vi "StatusPub0MQ.vi"() -> (0 "error":errorcluster)   [LabVIEW 2012]
uses:
  <vilib>/addons/zeromq/zmq_context.lvclass
  <vilib>/addons/zeromq/zmq_socket.lvclass
  <vilib>/addons/zeromq/socket_type.ctl
  Global_Telescopio.vi
  <vilib>/addons/zeromq/zeromq.lvlib
panel:
  out "pulledCommand":string
  out "status":string
  out "time string":string
  in  "panelSstop":bool
  # "TCSPD STATUS PUB"
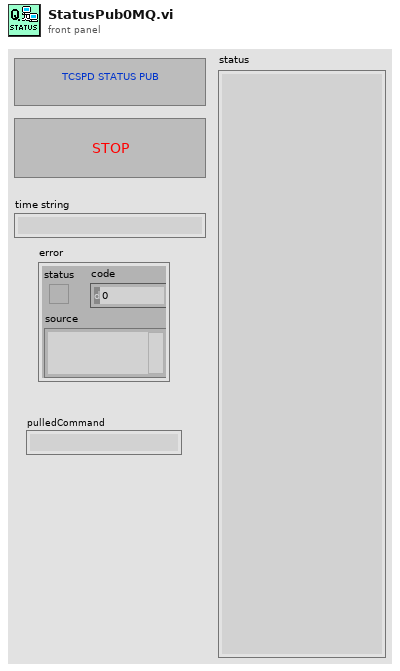
[diagram p1: front panel]
types:
  T1 = typedef "zeromq.lvlib/socket_type.ctl" = enum8{"ZMQ_PAIR", "ZMQ_PUB", "ZMQ_SUB", "ZMQ_REQ", "ZMQ_REP", "ZMQ_DEALER", "ZMQ_ROUTER", "ZMQ_PULL", "ZMQ_PUSH", "ZMQ_XPUB", "ZMQ_XSUB", "ZMQ_STREAM", "ZMQ_SERVER", "ZMQ_CLIENT", "ZMQ_RADIO", "ZMQ_DISH", "ZMQ_GATHER", "ZMQ_SCATTER", "ZMQ_DGRAM"}
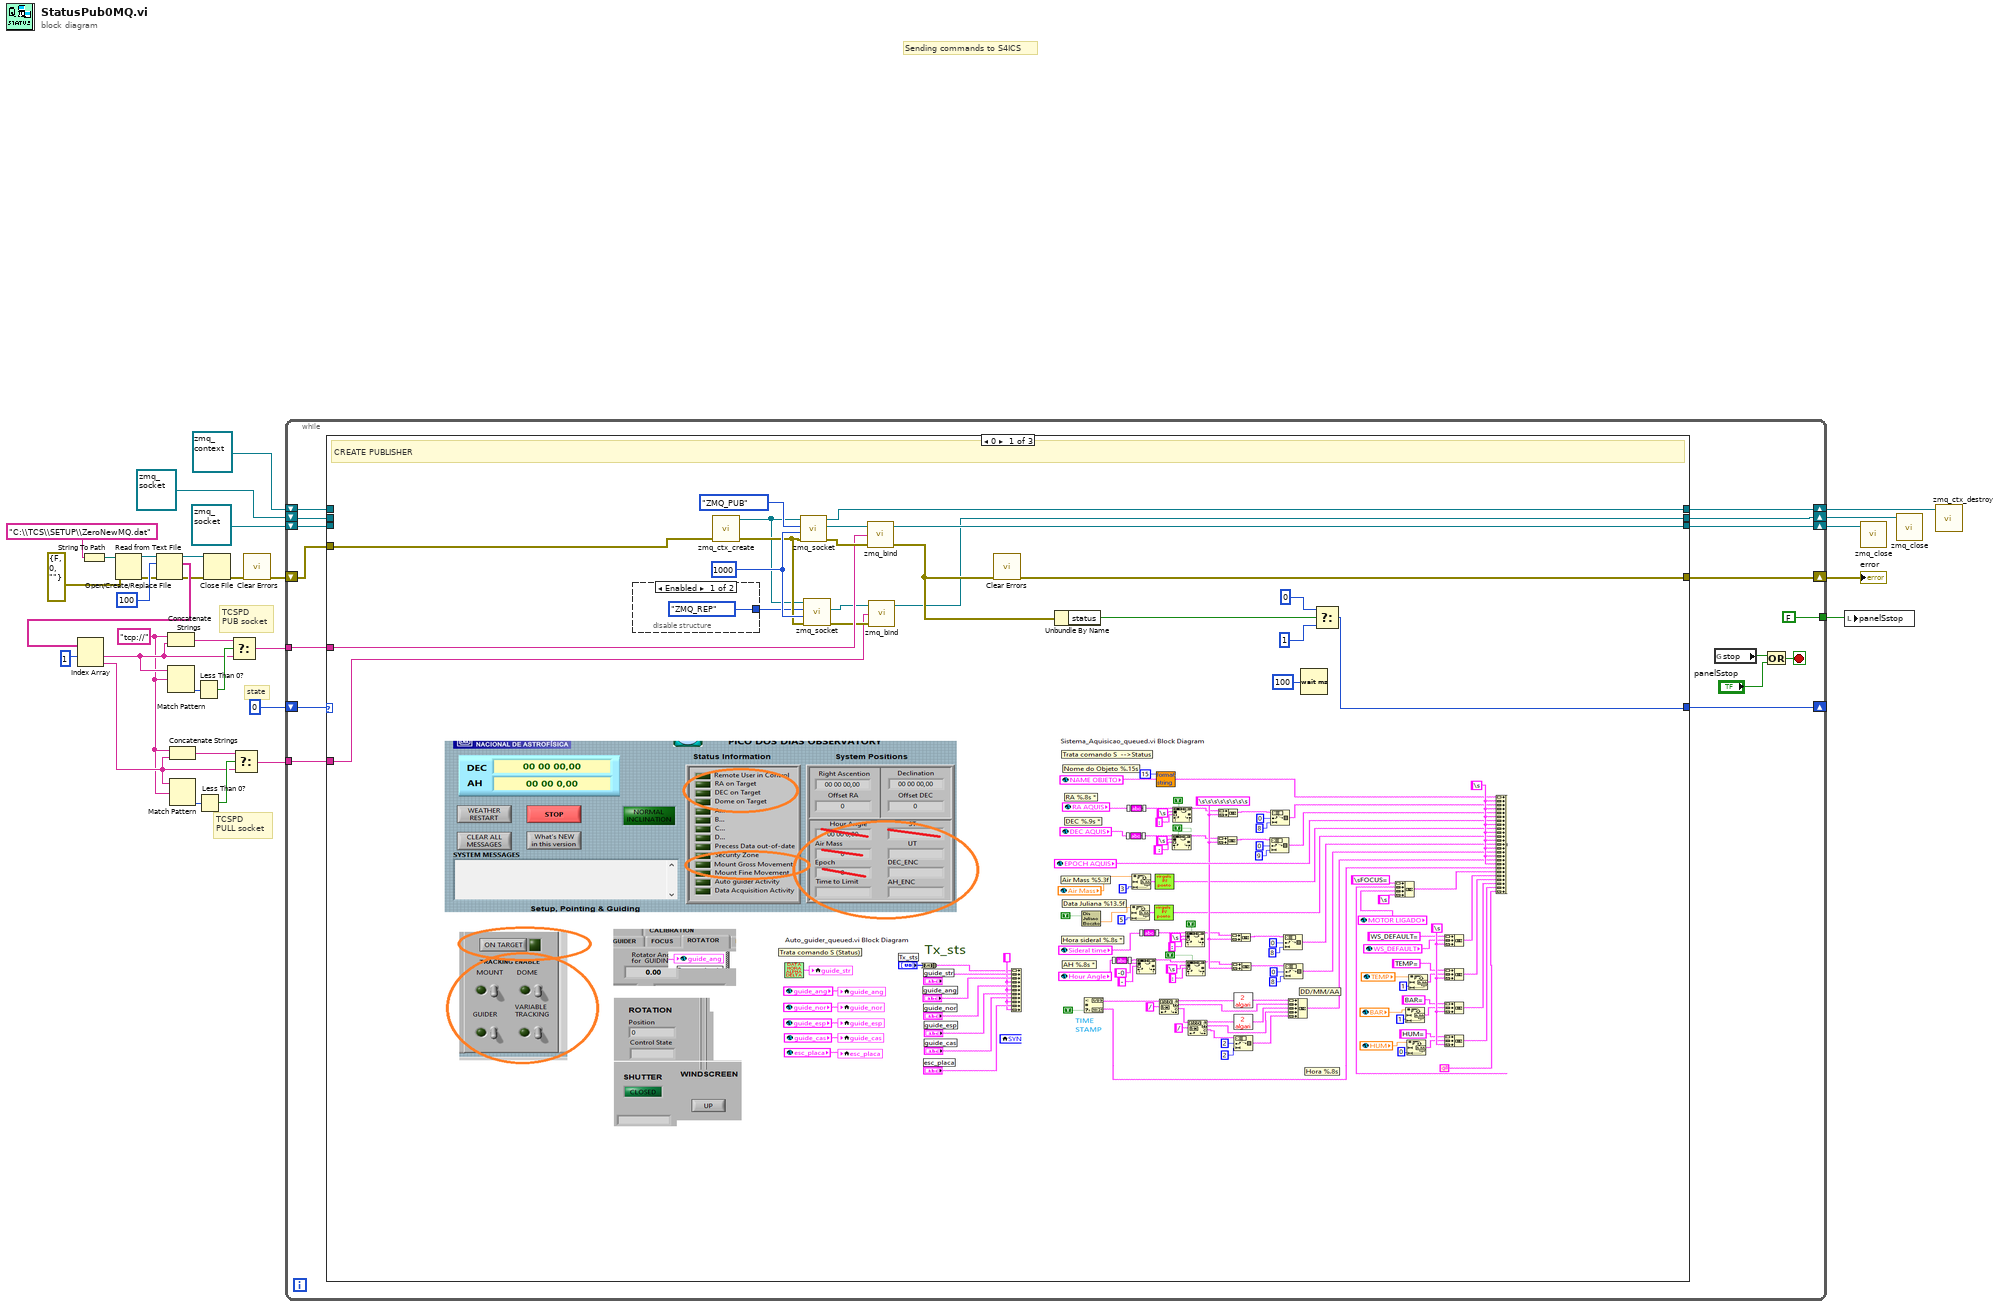
[diagram p0: block diagram]
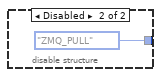
[diagram p2: hidden frame]
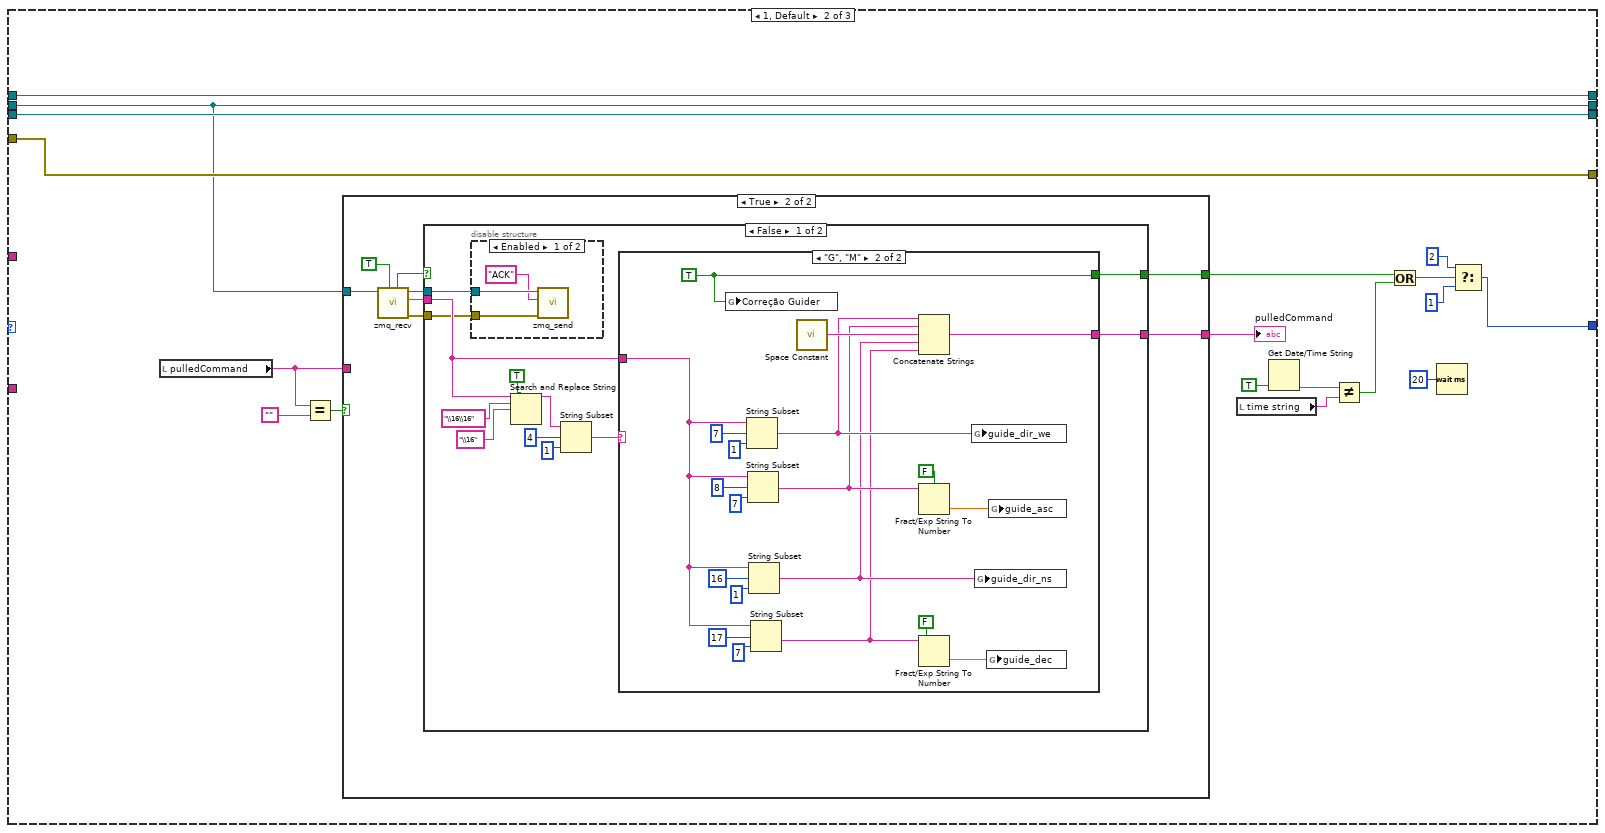
[diagram p3: hidden frame]
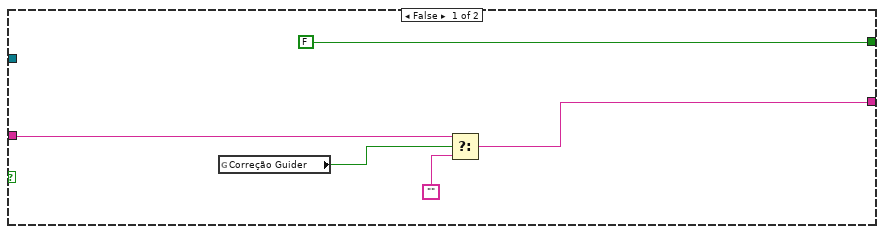
[diagram p4: hidden frame]
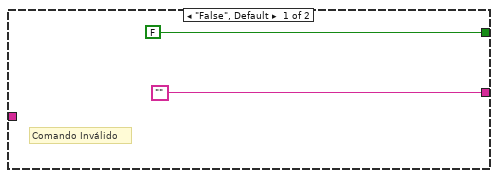
[diagram p6: hidden frame]
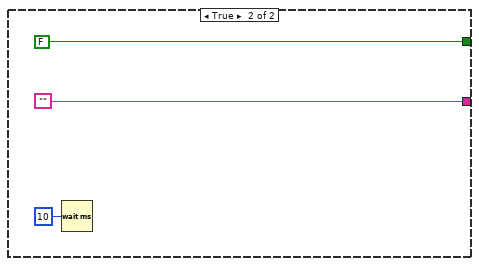
[diagram p7: hidden frame]
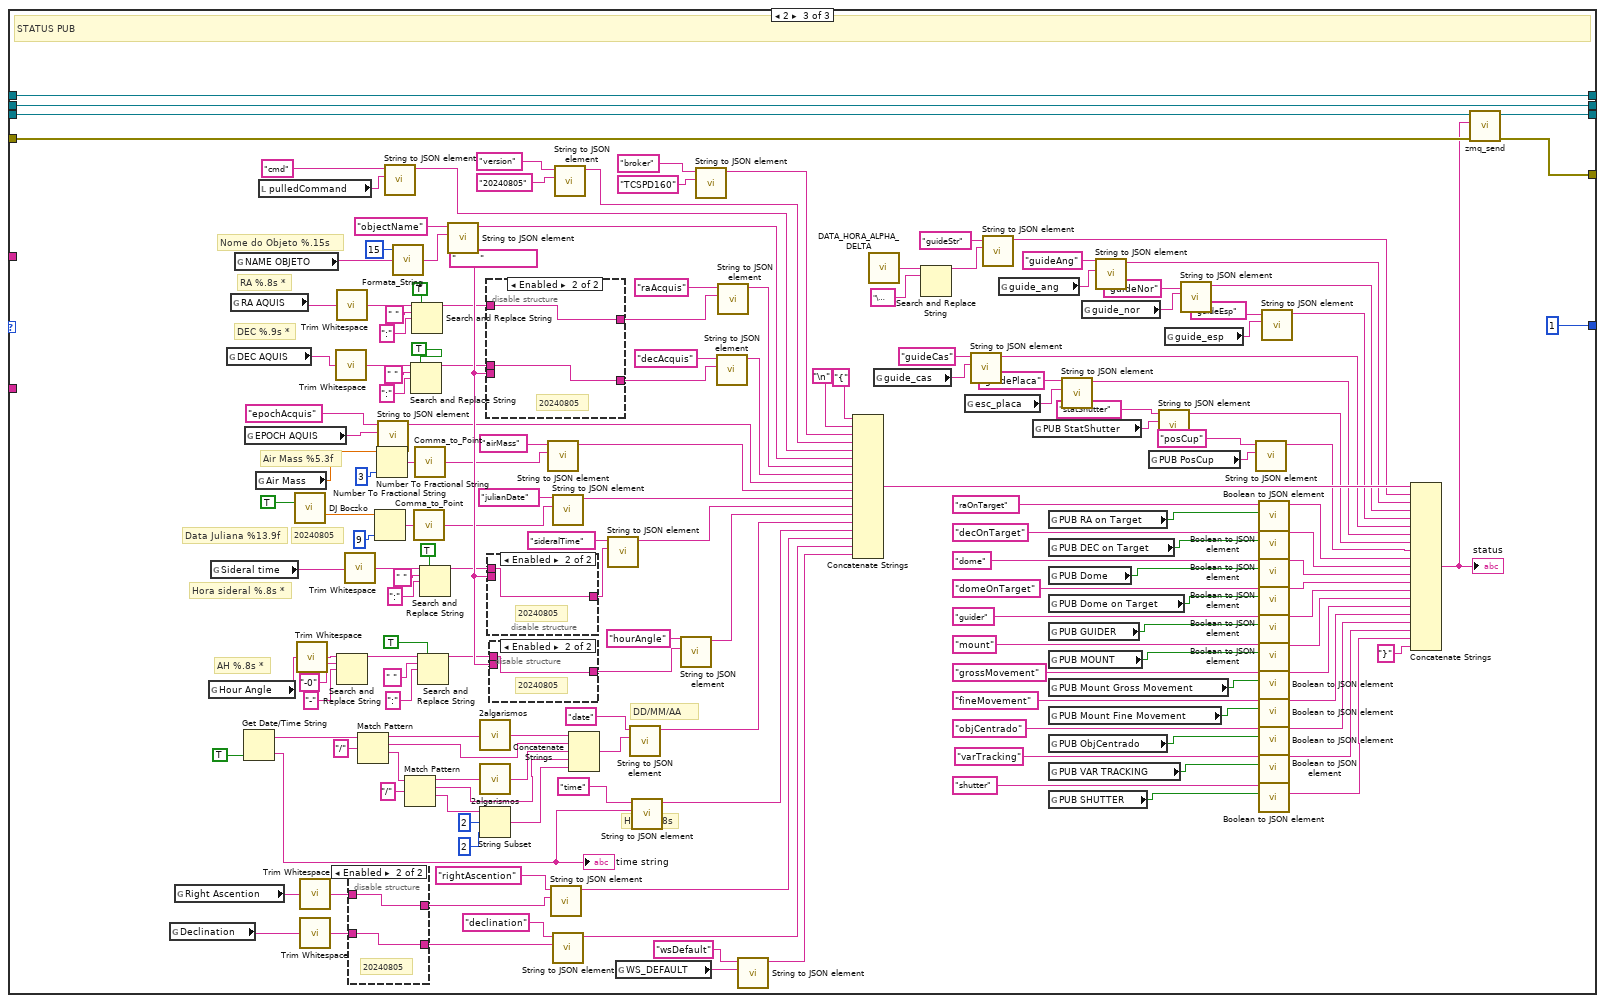
[diagram p8: hidden frame]
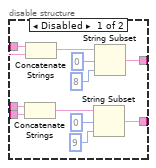
[diagram p9: hidden frame]
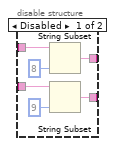
[diagram p10: hidden frame]
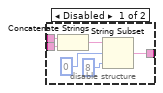
[diagram p11: hidden frame]
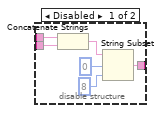
[diagram p12: hidden frame]
diagram:
  w2 = "tcp://"
  # "TCSPD\nPULL socket"
  # "TCSPD\nPUB socket"
  # "state"
  # "Sending commands to S4ICS"
  n1 = String To Path(string="C:\\TCS\\SETUP\\ZeroNewMQ.dat") -> (path=w31:path)
  n2 = Open/Create/Replace File(file path (use dialog)=w31, error in=errorcluster {"status"=FALSE, "code"=0, "source"=""}) -> (refnum out=w29:refnum<file>, error out=w22:errorcluster)  [unwired: 4 in, 1 out]
  n3 = Read from Text File(file (use dialog)=w29, count=100, error in=w22) -> (refnum out=w25:refnum<file>, text=w27:string[], error out=w19:errorcluster)  [unwired: 1 in, 1 out]
  n4 = Index Array(array=w27, index #1=1 ("index")) -> (element #1=w11:string, element #2=w3:string)  [unwired: 1 in]
  n5 = Concatenate Strings(w2, w11) -> (w13:string)
  n6 = Match Pattern(string=w11, regular expression=w2) -> (offset past match=w12:i32)  [unwired: 1 in, 3 out]
  n7 = Concatenate Strings(w2, w3) -> (w5:string)
  n8 = Match Pattern(string=w3, regular expression=w2) -> (offset past match=w6:i32)  [unwired: 1 in, 3 out]
  n9 = Less Than 0?(x=w12) -> (x < 0?=w14:bool)
  n10 = Less Than 0?(x=w6) -> (x < 0?=w4:bool)
  n11 = Close File(refnum=w25, error in=w19) -> (error out=w20:errorcluster)  [unwired: 1 out]
  n12 = Select(t=w13, s=w14, f=w11) -> (s? t:f=w10:string)
  n13 = Select(t=w5, s=w4, f=w3) -> (s? t:f=w1:string)
  n14 = call <vilib>:"Clear Errors.vi"("error in (no error)"=w20) -> ("error out"=w18:errorcluster)  [unwired: 6 in]
  n15 = while {
    shift-right: [w46] -> _
    shift-left: u16 0 -> [w48]
    tunnel: w10 -> [w44]
    shift-right: [w42] -> w16
    shift-left: refnum<class "zmq_socket.lvclass"> refnum ("socket out") -> [w43]
    shift-right: [w41] -> w21
    shift-left: refnum<class "zmq_context.lvclass"> refnum ("context out") -> [w40]
    tunnel: [FALSE] -> w15
    shift-right: [w37] -> w9
    shift-left: w18 -> [w47]
    shift-right: [w35] -> w7
    shift-left: refnum<class "zmq_socket.lvclass"> refnum ("socket out") -> [w34]
    tunnel: w1 -> [w33]
    stop <- w45 stop-if-true
    n16 = case shown="0" w48 {
      tunnel: w47 -> [w66 w87 w311]
      tunnel: [w68 w88 u16 1] -> w46
      tunnel: w44 -> [w59 _ _]
      tunnel: w43 -> [_ w86 w314]
      tunnel: [w58 w86 w313] -> w42
      tunnel: [w67 w84 w312] -> w41
      tunnel: w40 -> [_ w84 w312]
      tunnel: [w61 w87 w310] -> w37
      tunnel: [w50 w85 w309] -> w35
      tunnel: w34 -> [_ w85 w309]
      tunnel: w33 -> [w49 _ _]
      frame 0 {
        w56 = 1000 ("linger (ms)")
        # "CREATE PUBLISHER"
        n17 = disable-structure shown="Enabled" {
          disable-tunnel: [socket_type."ZMQ_REP" ("socket type") socket_type."ZMQ_PULL" ("socket type")] -> w53
          frame Enabled {
          }
          frame Disabled {
          }
        }
        n18 = call <vilib>:"zmq_ctx_create.vi"("error in"=w66) -> ("error out"=w55:errorcluster, "context out"=w54:refnum<class "zmq_context.lvclass">)  [unwired: 3 in]
        n19 = call <vilib>:"zmq_socket.vi"("error in"=w55, "linger (ms)"=w56, "socket type"=socket_type."ZMQ_PUB", "context in"=w54) -> ("error out"=w63:errorcluster, "socket out"=w64:refnum<class "zmq_socket.lvclass">, "context out"=w67:refnum<class "zmq_context.lvclass">)  [unwired: 1 in]
        n20 = call <vilib>:"zmq_socket.vi"("error in"=w55, "linger (ms)"=w56, "socket type"=w53, "context in"=w54) -> ("error out"=w51:errorcluster, "socket out"=w52:refnum<class "zmq_socket.lvclass">)  [unwired: 1 in, 1 out]
        n21 = call <vilib>:"zmq_bind.vi"("error in"=w63, "endpoint"=w59, "socket in"=w64) -> ("error out"=w60:errorcluster, "socket out"=w58:refnum<class "zmq_socket.lvclass">)  [unwired: 1 in]
        n22 = call <vilib>:"zmq_bind.vi"("error in"=w51, "endpoint"=w49, "socket in"=w52) -> ("socket out"=w50:refnum<class "zmq_socket.lvclass">)  [unwired: 1 in, 1 out]
        n23 = call <vilib>:"Clear Errors.vi"("error in (no error)"=w60) -> ("error out"=w61:errorcluster)  [unwired: 6 in]
        n24 = Unbundle By Name(w60) -> ("status"=w57:bool)
        n25 = Wait (ms)(milliseconds to wait=u32 100) -> ()  [unwired: 1 out]
        n26 = Select(t=u16 0, s=w57, f=u16 1) -> (s? t:f=w68:u16)
      }
      frame 1, Default {
        n27 = local read "pulledCommand"() -> (w76:string)
        n28 = Equal?(x=w76, y="") -> (x = y?=w78:bool)
        n29 = case shown="True" w78 {
          tunnel: w85 -> [_ w103]
          tunnel: [w91 w100] -> w73
          tunnel: w76 -> [w93 _]
          tunnel: [FALSE w99] -> w75
          frame False {
            n30 = global read "Global_Telescopio.vi" "Correção Guider"() -> (w94:bool)
            n31 = Select(t=w93, s=w94, f="") -> (s? t:f=w91:string)
          }
          frame True {
            n32 = call <vilib>:"zmq_recv.vi"("no block? (F)"=TRUE, "socket in"=w103) -> ("error out"=w96:errorcluster, "data"=w101:string, "socket out"=w97:refnum<class "zmq_socket.lvclass">, "timeout?"=w98:bool)  [unwired: 3 in, 1 out]
            n33 = case shown="False" w98 {
              tunnel: w101 -> [w108 _]
              tunnel: [w107 ""] -> w100
              tunnel: [w106 FALSE] -> w99
              tunnel: w97 -> [w105 _]
              tunnel: w96 -> [w104 _]
              frame False {
                n34 = disable-structure shown="Enabled" {
                  disable-tunnel: w105 -> [w118 _]
                  disable-tunnel: w104 -> [w117 _]
                  frame Enabled {
                    n35 = call <vilib>:"zmq_send.vi"("error in"=w117, "data"="ACK", "socket in"=w118) -> ()  [unwired: 4 in, 2 out]
                  }
                  frame Disabled {
                  }
                }
                n36 = Search and Replace String(replace all?=TRUE ("replace all? (F)"), input string=w108, search string="\\16\\16", replace string="\\16" ("replace string (\"\")")) -> (result string=w110:string)  [unwired: 4 in, 3 out]
                n37 = String Subset(string=w110, offset (0)=4, length (rest)=1 ("length (rest)")) -> (substring=w109:string)
                n38 = case shown="\"G\", \"M\"" w109 {
                  tunnel: w108 -> [_ w127]
                  tunnel: ["" w121] -> w107
                  tunnel: [FALSE w128] -> w106
                  frame "False", Default {
                    # "Comando Inválido"
                  }
                  frame "G", "M" {
                    w128 = TRUE ("replace all? (F)")
                    n39 = global write "Global_Telescopio.vi" "Correção Guider"(w128) -> ()
                    n40 = String Subset(string=w127, offset (0)=7, length (rest)=1 ("length (rest)")) -> (substring=w125:string)
                    n41 = String Subset(string=w127, offset (0)=8, length (rest)=7 ("length (rest)")) -> (substring=w124:string)
                    n42 = String Subset(string=w127, offset (0)=16, length (rest)=1 ("length (rest)")) -> (substring=w123:string)
                    n43 = String Subset(string=w127, offset (0)=17, length (rest)=7 ("length (rest)")) -> (substring=w122:string)
                    n44 = call <vilib>:"Space Constant.vi"() -> ("String"=w126:string)
                    n45 = Concatenate Strings(w125, w124, w126, w123, w122) -> (w121:string)
                    n46 = Fract/Exp String To Number(use system decimal point (T)=FALSE, string=w124) -> (number=w139:dbl)  [unwired: 2 in, 1 out]
                    n47 = Fract/Exp String To Number(use system decimal point (T)=FALSE, string=w122) -> (number=w140:dbl)  [unwired: 2 in, 1 out]
                    n48 = global write "Global_Telescopio.vi" "guide_dir_we"(w125) -> ()
                    n49 = global write "Global_Telescopio.vi" "guide_dir_ns"(w123) -> ()
                    n50 = global write "Global_Telescopio.vi" "guide_dec"(w140) -> ()
                    n51 = global write "Global_Telescopio.vi" "guide_asc"(w139) -> ()
                  }
                }
              }
              frame True {
                n52 = Wait (ms)(milliseconds to wait=u32 10) -> ()  [unwired: 1 out]
              }
            }
          }
        }
        "pulledCommand" <- w73
        n53 = local read "time string"() -> (w79:string)
        n54 = Get Date/Time String(want seconds? (F)=TRUE) -> (time string=w80:string)  [unwired: 2 in, 1 out]
        n55 = Not Equal?(x=w80, y=w79) -> (x != y?=w82:bool)
        n56 = Or(x=w75, y=w82) -> (x .or. y?=w83:bool)
        n57 = Wait (ms)(milliseconds to wait=u32 20) -> ()  [unwired: 1 out]
        n58 = Select(t=u16 2, s=w83, f=u16 1) -> (s? t:f=w88:u16)
      }
      frame 2 {
        w285 = "        " ("string")
        # "20240805"
        # "Hora %.8s"
        # "DD/MM/AA"
        # "AH %.8s *"
        # "Hora sideral %.8s *"
        # "Data Juliana %13.9f"
        # "Air Mass %5.3f"
        # "DEC %.9s *"
        # "RA %.8s *"
        # "Nome do Objeto %.15s"
        # "STATUS PUB"
        n59 = global read "Global_Telescopio.vi" "Declination"() -> (w170:string)
        n60 = global read "Global_Telescopio.vi" "Right Ascention"() -> (w168:string)
        n61 = global read "Global_Telescopio.vi" "Hour Angle"() -> (w308:string)
        n62 = global read "Global_Telescopio.vi" "Sideral time"() -> (w280:string)
        n63 = global read "Global_Telescopio.vi" "DEC AQUIS"() -> (w269:string)
        n64 = global read "Global_Telescopio.vi" "RA AQUIS"() -> (w259:string)
        n65 = global read "Global_Telescopio.vi" "NAME OBJETO"() -> (w302:string)
        n66 = Get Date/Time String(want seconds? (F)=TRUE) -> (date string=w318:string, time string=w316:string)  [unwired: 2 in]
        "time string" <- w316
        n67 = global read "Global_Telescopio.vi" "EPOCH AQUIS"() -> (w248:string)
        n68 = global read "Global_Telescopio.vi" "Air Mass"() -> (w301:dbl)
        n69 = local read "pulledCommand"() -> (w152:string)
        n70 = call "DJ Boczko.vi"("TRUE = Hora Local\nFALSE = UT"=TRUE ("TRUE = Hora Local\nFALSE = UT")) -> ("Dia Juliano"=w274:dbl)  [unwired: 6 in, 8 out]
        n71 = call <vilib>:"Trim Whitespace.vi"("string"=w308) -> ("trimmed string"=w307:string)  [unwired: 1 in]
        n72 = call <vilib>:"Trim Whitespace.vi"("string"=w168) -> ("trimmed string"=w167:string)  [unwired: 1 in]
        n73 = call <vilib>:"Trim Whitespace.vi"("string"=w170) -> ("trimmed string"=w169:string)  [unwired: 1 in]
        n74 = call <vilib>:"Trim Whitespace.vi"("string"=w269) -> ("trimmed string"=w268:string)  [unwired: 1 in]
        n75 = call <vilib>:"Trim Whitespace.vi"("string"=w259) -> ("trimmed string"=w260:string)  [unwired: 1 in]
        n76 = Search and Replace String(input string=w307, search string="-0", replace string="-" ("replace string (\"\")")) -> (result string=w306:string)  [unwired: 5 in, 3 out]
        n77 = call <vilib>:"Trim Whitespace.vi"("string"=w280) -> ("trimmed string"=w279:string)  [unwired: 1 in]
        n78 = disable-structure shown="Enabled" {
          disable-tunnel: w169 -> [w337 w338]
          disable-tunnel: w167 -> [w335 w339]
          disable-tunnel: [w334 w339] -> w161
          disable-tunnel: [w333 w338] -> w160
          frame Disabled {
            n79 = String Subset(string=w335, length (rest)=8 ("length (rest)")) -> (substring=w334:string)  [unwired: 1 in]
            n80 = String Subset(string=w337, length (rest)=9 ("length (rest)")) -> (substring=w333:string)  [unwired: 1 in]
          }
          frame Enabled {
            # "20240805"
          }
        }
        n81 = Match Pattern(string=w318, regular expression="/") -> (before substring=w289:string, match substring=w295:string, after substring=w288:string)  [unwired: 1 in, 1 out]
        n82 = Number To Fractional String(number=w274, precision (6)=i16 9) -> (F-format string=w275:string)  [unwired: 2 in]
        n83 = Number To Fractional String(number=w301, precision (6)=i16 3) -> (F-format string=w272:string)  [unwired: 2 in]
        n84 = call "String to JSON element.vi"("value"=w248, "keyword"="epochAcquis") -> ("JSON element"=w247:string)  [unwired: 8 in, 1 out]
        n85 = call "String to JSON element.vi"("value"=w152, "keyword"="cmd") -> ("JSON element"=w147:string)  [unwired: 8 in, 1 out]
        n86 = call "Formata_String.vi"("entrada"=w302, "Num de Caracteres"=15) -> ("saida"=w257:string)  [unwired: 3 in]
        n87 = Match Pattern(string=w288, regular expression="/") -> (before substring=w290:string, match substring=w297:string, after substring=w291:string)  [unwired: 1 in, 1 out]
        n88 = Search and Replace String(replace all?=TRUE ("replace all? (F)"), input string=w268, search string=" ", replace string=":" ("replace string (\"\")")) -> (result string=w265:string)  [unwired: 4 in, 3 out]
        n89 = Search and Replace String(replace all?=TRUE ("replace all? (F)"), input string=w260, search string=" ", replace string=":" ("replace string (\"\")")) -> (result string=w264:string)  [unwired: 4 in, 3 out]
        n90 = call "Comma_to_Point.vi"("Lat_A"=w275) -> ("Saída"=w242:string)
        n91 = call "Comma_to_Point.vi"("Lat_A"=w272) -> ("Saída"=w246:string)
        n92 = Search and Replace String(replace all?=TRUE ("replace all? (F)"), input string=w306, search string=" ", replace string=":" ("replace string (\"\")")) -> (result string=w284:string)  [unwired: 4 in, 3 out]
        n93 = Search and Replace String(replace all?=TRUE ("replace all? (F)"), input string=w279, search string=" ", replace string=":" ("replace string (\"\")")) -> (result string=w276:string)  [unwired: 4 in, 3 out]
        n94 = call "String to JSON element.vi"("value"=w257, "keyword"="objectName") -> ("JSON element"=w256:string)  [unwired: 8 in, 1 out]
        n95 = call "2algarismos.vi"("entrada"=w289) -> ("saida"=w294:string)
        n96 = call "2algarismos.vi"("entrada"=w290) -> ("saida"=w296:string)
        n97 = String Subset(string=w291, offset (0)=2, length (rest)=2 ("length (rest)")) -> (substring=w298:string)
        n98 = disable-structure shown="Enabled" {
          disable-tunnel: w285 -> [w329 _]
          disable-tunnel: w265 -> [w326 w331]
          disable-tunnel: w264 -> [w323 w330]
          disable-tunnel: [w320 w330] -> w255
          disable-tunnel: [w319 w331] -> w252
          frame Disabled {
            n99 = Concatenate Strings(w326, w329) -> (w325:string)
            n100 = Concatenate Strings(w323, w329) -> (w324:string)
            n101 = String Subset(string=w325, offset (0)=0, length (rest)=9 ("length (rest)")) -> (substring=w319:string)
            n102 = String Subset(string=w324, offset (0)=0, length (rest)=8 ("length (rest)")) -> (substring=w320:string)
          }
          frame Enabled {
            # "20240805"
          }
        }
        n103 = disable-structure shown="Enabled" {
          disable-tunnel: w285 -> [w352 _]
          disable-tunnel: w276 -> [w349 w353]
          disable-tunnel: [w347 w353] -> w239
          frame Disabled {
            n104 = Concatenate Strings(w349, w352) -> (w348:string)
            n105 = String Subset(string=w348, offset (0)=0, length (rest)=8 ("length (rest)")) -> (substring=w347:string)
          }
          frame Enabled {
            # "20240805"
          }
        }
        n106 = disable-structure shown="Enabled" {
          disable-tunnel: w285 -> [w345 _]
          disable-tunnel: w284 -> [w343 w346]
          disable-tunnel: [w340 w346] -> w236
          frame Disabled {
            n107 = Concatenate Strings(w343, w345) -> (w344:string)
            n108 = String Subset(string=w344, offset (0)=0, length (rest)=8 ("length (rest)")) -> (substring=w340:string)
          }
          frame Enabled {
            # "20240805"
          }
        }
        n109 = call "String to JSON element.vi"("value"=w246, "keyword"="airMass") -> ("JSON element"=w244:string)  [unwired: 8 in, 1 out]
        n110 = call "String to JSON element.vi"("value"=w161, "keyword"="rightAscention") -> ("JSON element"=w159:string)  [unwired: 8 in, 1 out]
        n111 = call "String to JSON element.vi"("value"=w242, "keyword"="julianDate") -> ("JSON element"=w241:string)  [unwired: 8 in, 1 out]
        n112 = call "String to JSON element.vi"("value"=w160, "keyword"="declination") -> ("JSON element"=w158:string)  [unwired: 8 in, 1 out]
        n113 = call "String to JSON element.vi"("value"="20240805", "keyword"="version") -> ("JSON element"=w148:string)  [unwired: 8 in, 1 out]
        n114 = Concatenate Strings(w294, w295, w296, w297, w298) -> (w233:string)
        n115 = call "String to JSON element.vi"("value"=w239, "keyword"="sideralTime") -> ("JSON element"=w238:string)  [unwired: 8 in, 1 out]
        n116 = global read "Global_Telescopio.vi" "WS_DEFAULT"() -> (w145:string)
        n117 = call "String to JSON element.vi"("value"=w233, "keyword"="date") -> ("JSON element"=w232:string)  [unwired: 8 in, 1 out]
        n118 = call "String to JSON element.vi"("value"=w316, "keyword"="time") -> ("JSON element"=w230:string)  [unwired: 8 in, 1 out]
        n119 = call "String to JSON element.vi"("value"=w236, "keyword"="hourAngle") -> ("JSON element"=w235:string)  [unwired: 8 in, 1 out]
        n120 = call "String to JSON element.vi"("value"="TCSPD160", "keyword"="broker") -> ("JSON element"=w149:string)  [unwired: 8 in, 1 out]
        n121 = call "String to JSON element.vi"("value"=w252, "keyword"="decAcquis") -> ("JSON element"=w250:string)  [unwired: 8 in, 1 out]
        n122 = call "String to JSON element.vi"("value"=w255, "keyword"="raAcquis") -> ("JSON element"=w253:string)  [unwired: 8 in, 1 out]
        n123 = call "String to JSON element.vi"("value"=w145, "keyword"="wsDefault") -> ("JSON element"=w144:string)  [unwired: 8 in, 1 out]
        n124 = Concatenate Strings("{", "\n", w149, w148, w147, w256, w253, w250, w247, w244, w241, w238, w235, w232, w230, w159, w158, w144) -> (w192:string)
        n125 = call "DATA_HORA_ALPHA_DELTA.vi"() -> ("SAIDA"=w166:string)  [unwired: 2 in]
        n126 = global read "Global_Telescopio.vi" "guide_cas"() -> (w221:string)
        n127 = Search and Replace String(input string=w166, search string="\u0000") -> (result string=w164:string)  [unwired: 6 in, 3 out]
        n128 = global read "Global_Telescopio.vi" "esc_placa"() -> (w219:string)
        n129 = call "String to JSON element.vi"("value"=w221, "keyword"="guideCas") -> ("JSON element"=w187:string)  [unwired: 8 in, 1 out]
        n130 = call "String to JSON element.vi"("value"=w164, "keyword"="guideStr") -> ("JSON element"=w191:string)  [unwired: 8 in, 1 out]
        n131 = global read "Global_Telescopio.vi" "guide_ang"() -> (w227:string)
        n132 = global read "Global_Telescopio.vi" "PUB StatShutter"() -> (w196:string)
        n133 = global read "Global_Telescopio.vi" "PUB RA on Target"() -> (w208:bool)
        n134 = global read "Global_Telescopio.vi" "PUB DEC on Target"() -> (w207:bool)
        n135 = global read "Global_Telescopio.vi" "PUB Dome"() -> (w206:bool)
        n136 = global read "Global_Telescopio.vi" "PUB Dome on Target"() -> (w205:bool)
        n137 = global read "Global_Telescopio.vi" "PUB GUIDER"() -> (w204:bool)
        n138 = global read "Global_Telescopio.vi" "PUB MOUNT"() -> (w203:bool)
        n139 = global read "Global_Telescopio.vi" "PUB Mount Gross Movement"() -> (w202:bool)
        n140 = global read "Global_Telescopio.vi" "PUB Mount Fine Movement"() -> (w201:bool)
        n141 = global read "Global_Telescopio.vi" "PUB ObjCentrado"() -> (w200:bool)
        n142 = global read "Global_Telescopio.vi" "PUB VAR TRACKING"() -> (w199:bool)
        n143 = global read "Global_Telescopio.vi" "PUB SHUTTER"() -> (w197:bool)
        n144 = call "String to JSON element.vi"("value"=w219, "keyword"="guidePlaca") -> ("JSON element"=w186:string)  [unwired: 8 in, 1 out]
        n145 = global read "Global_Telescopio.vi" "guide_nor"() -> (w225:string)
        n146 = call "String to JSON element.vi"("value"=w227, "keyword"="guideAng") -> ("JSON element"=w190:string)  [unwired: 8 in, 1 out]
        n147 = global read "Global_Telescopio.vi" "PUB PosCup"() -> (w195:string)
        n148 = call "String to JSON element.vi"("value"=w196, "keyword"="statShutter") -> ("JSON element"=w185:string)  [unwired: 8 in, 1 out]
        n149 = global read "Global_Telescopio.vi" "guide_esp"() -> (w223:string)
        n150 = call "String to JSON element.vi"("value"=w225, "keyword"="guideNor") -> ("JSON element"=w189:string)  [unwired: 8 in, 1 out]
        n151 = call "String to JSON element.vi"("value"=w195, "keyword"="posCup") -> ("JSON element"=w184:string)  [unwired: 8 in, 1 out]
        n152 = call "Boolean to JSON element.vi"("boolean"=w208, "keyword"="raOnTarget") -> ("JSON element"=w183:string)  [unwired: 8 in, 1 out]
        n153 = call "Boolean to JSON element.vi"("boolean"=w207, "keyword"="decOnTarget") -> ("JSON element"=w182:string)  [unwired: 8 in, 1 out]
        n154 = call "Boolean to JSON element.vi"("boolean"=w206, "keyword"="dome") -> ("JSON element"=w181:string)  [unwired: 8 in, 1 out]
        n155 = call "Boolean to JSON element.vi"("boolean"=w205, "keyword"="domeOnTarget") -> ("JSON element"=w180:string)  [unwired: 8 in, 1 out]
        n156 = call "Boolean to JSON element.vi"("boolean"=w204, "keyword"="guider") -> ("JSON element"=w179:string)  [unwired: 8 in, 1 out]
        n157 = call "Boolean to JSON element.vi"("boolean"=w203, "keyword"="mount") -> ("JSON element"=w178:string)  [unwired: 8 in, 1 out]
        n158 = call "Boolean to JSON element.vi"("boolean"=w202, "keyword"="grossMovement") -> ("JSON element"=w177:string)  [unwired: 8 in, 1 out]
        n159 = call "Boolean to JSON element.vi"("boolean"=w201, "keyword"="fineMovement") -> ("JSON element"=w176:string)  [unwired: 8 in, 1 out]
        n160 = call "Boolean to JSON element.vi"("boolean"=w200, "keyword"="objCentrado") -> ("JSON element"=w175:string)  [unwired: 8 in, 1 out]
        n161 = call "Boolean to JSON element.vi"("boolean"=w199, "keyword"="varTracking") -> ("JSON element"=w174:string)  [unwired: 8 in, 1 out]
        n162 = call "Boolean to JSON element.vi"("boolean"=w197, "keyword"="shutter") -> ("JSON last element"=w173:string)  [unwired: 8 in, 1 out]
        n163 = call "String to JSON element.vi"("value"=w223, "keyword"="guideEsp") -> ("JSON element"=w188:string)  [unwired: 8 in, 1 out]
        n164 = Concatenate Strings(w192, w191, w190, w189, w188, w187, w186, w185, w184, w183, w182, w181, w180, w179, w178, w177, w176, w175, w174, w173, "}") -> (w171:string)
        "status" <- w171
        n165 = call <vilib>:"zmq_send.vi"("error in"=w311, "data"=w171, "socket in"=w314) -> ("error out"=w310:errorcluster, "socket out"=w313:refnum<class "zmq_socket.lvclass">)  [unwired: 4 in]
      }
    }
    n166 = global read "Global_Telescopio.vi" "stop"() -> (w36:bool)
    n167 = Or(x=w36, y="panelSstop") -> (x .or. y?=w45:bool)
  }
  "error" <- w9
  n168 = local write "panelSstop"(w15) -> ()
  n169 = call <vilib>:"zmq_close.vi"("socket"=w16) -> ()  [unwired: 4 in, 1 out]
  n170 = call <vilib>:"zmq_close.vi"("socket"=w7) -> ()  [unwired: 4 in, 1 out]
  n171 = call <vilib>:"zmq_ctx_destroy.vi"("context in"=w21) -> ()  [unwired: 4 in, 1 out]
